vi "1. VI PRINCIPAL DDP GPE.vi"() -> ()   [LabVIEW 2019]
panel:
  out "Timeout":bool
  in  "Stop Button":bool
  in  "Menú":enum32{"Edición", "Reporte"}(tab)
  in  "Tab Control":T1(tab)
  out "Horizontal Pointer Slide 1":dbl
  in  "Umbralado":dbl(slide) scale=0.0..255.0
  in  "Umbralado Invertido":dbl(slide) scale=0.0..255.0
  out "Umbralado Invertido 2":dbl
  in  "Prewitt":dbl(slide) scale=0.0..10.0
  in  "Sobel":dbl(slide) scale=0.0..255.0
  out "Sobel Ind":dbl
  out "Prewitt Ind":dbl
  out "Filtro 2 Ind":dbl
  out "Filtro 1 Ind":dbl
  in  "Filtro 2":dbl(slide) scale=0.0..10.0
  in  "Filtro 1":dbl(slide) scale=0.0..10.0
  in  "+":bool
  in  "-":bool
  out "+ 2":bool
  out "- 2":bool
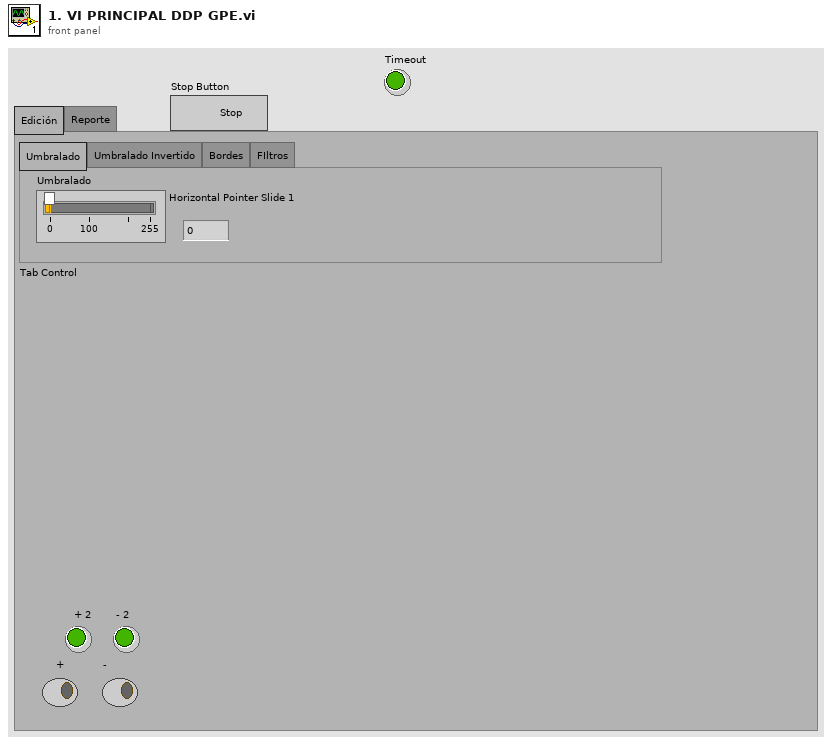
[diagram p1: front panel]
types:
  T1 = enum32{"Umbralado", "Umbralado Invertido", "Bordes", "FIltros"}
  T2 = cluster{"Umbralado":dbl, "Umbralado Invertido":dbl, "Filtro 1":dbl, "Filtro 2":dbl, "Sobel":dbl, "Prewitt":dbl}
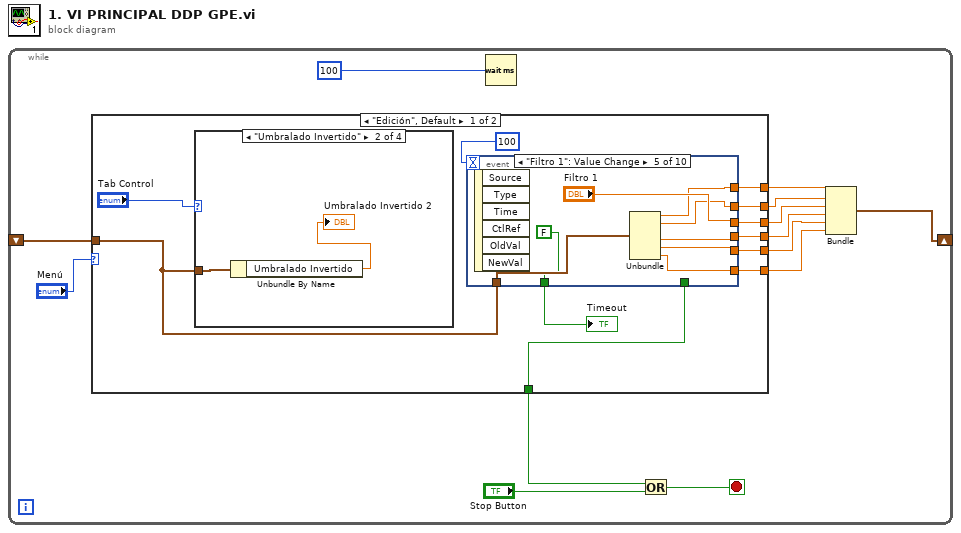
[diagram p0: block diagram]
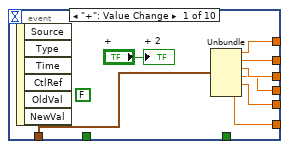
[diagram p2: hidden frame]
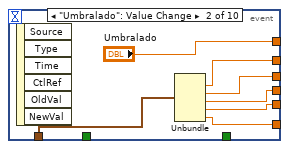
[diagram p3: hidden frame]
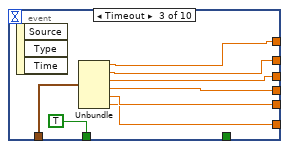
[diagram p4: hidden frame]
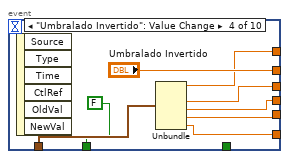
[diagram p5: hidden frame]
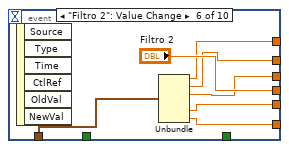
[diagram p6: hidden frame]
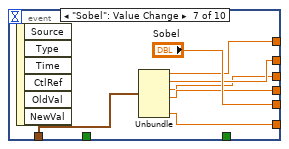
[diagram p7: hidden frame]
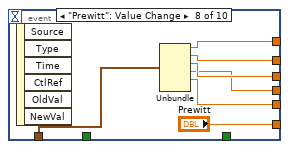
[diagram p8: hidden frame]
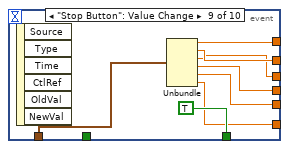
[diagram p9: hidden frame]
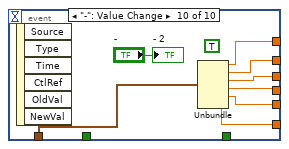
[diagram p10: hidden frame]
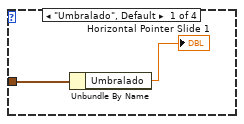
[diagram p11: hidden frame]
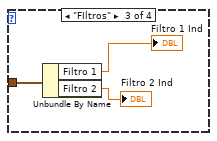
[diagram p12: hidden frame]
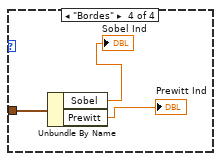
[diagram p13: hidden frame]
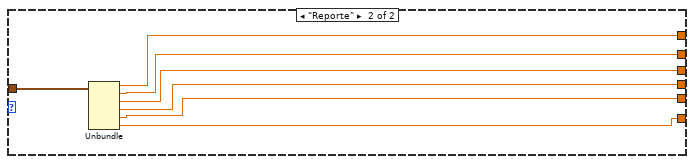
[diagram p14: hidden frame]
diagram:
  n1 = while {
    shift-right: [w5] -> _
    shift-left: _ -> [w8]
    stop <- w11 stop-if-true
    n2 = case shown="\"Edición\", Default" "Menú" {
      tunnel: [w23 _] -> w9
      tunnel: [w21 w115] -> w6
      tunnel: [w20 w116] -> w7
      tunnel: w8 -> [w15 w117]
      tunnel: [w19 w114] -> w4
      tunnel: [w18 w113] -> w3
      tunnel: [w17 w112] -> w2
      tunnel: [w16 w111] -> w1
      frame "Edición", Default {
        n3 = case shown="\"Umbralado Invertido\"" "Tab Control" {
          tunnel: w15 -> [w102 w104 w107 w110]
          frame "Umbralado", Default {
            n4 = Unbundle By Name(w102) -> ("Umbralado"=→"Horizontal Pointer Slide 1":dbl)
          }
          frame "Umbralado Invertido" {
            n5 = Unbundle By Name(w104) -> ("Umbralado Invertido"=→"Umbralado Invertido 2":dbl)
          }
          frame "FIltros" {
            n6 = Unbundle By Name(w107) -> ("Filtro 1"=→"Filtro 1 Ind":dbl, "Filtro 2"=→"Filtro 2 Ind":dbl)
          }
          frame "Bordes" {
            n7 = Unbundle By Name(w110) -> ("Sobel"=→"Sobel Ind":dbl, "Prewitt"=→"Prewitt Ind":dbl)
          }
        }
        n8 = event shown="[4] \"Filtro 1\": Value Change" {
          selector: _ -> [_ _ _ _ _ _ _ _ _ _]
          dyn-events: _ -> [_ _ _ _ _ _ _ _ _ _]
          timeout: 100 -> [_ _ _ _ _ _ _ _ _ _]
          tunnel: [_ _ _ _ _ _ _ _ TRUE _] -> w23
          tunnel: [w29 w37 w45 "Umbralado Invertido" w60 w67 w72 w81 w89 w97] -> w21
          tunnel: [w30 "Umbralado" w46 w53 w61 w68 w74 w82 w90 w98] -> w20
          tunnel: [w28 w36 w44 w52 "Filtro 1" w66 w71 w80 w88 w96] -> w19
          tunnel: [w27 w35 w43 w51 w59 "Filtro 2" w73 w79 w87 w95] -> w18
          tunnel: [w26 w34 w42 w50 w58 w65 "Sobel" w78 w86 w94] -> w17
          tunnel: [w25 w33 w41 w49 w57 w64 w75 "Prewitt" w85 w93] -> w16
          tunnel: w15 -> [w31 w38 w47 w54 w62 w69 w76 w83 w91 w99]
          tunnel: [_ _ TRUE ("Timeout") FALSE FALSE _ _ _ _ _] -> w14
          event "+": Value Change {
            (unwired) FALSE
            n9 = event-data() -> ()  [unwired: 1 in, 6 out]
            n10 = Unbundle(w31) -> ("Umbralado"=w30:dbl, "Umbralado Invertido"=w29:dbl, "Filtro 1"=w28:dbl, "Filtro 2"=w27:dbl, "Sobel"=w26:dbl, "Prewitt"=w25:dbl)
            "+ 2" <- "+"
          }
          event "Umbralado": Value Change {
            n11 = event-data() -> ()  [unwired: 1 in, 6 out]
            n12 = Unbundle(w38) -> ("Umbralado Invertido"=w37:dbl, "Filtro 1"=w36:dbl, "Filtro 2"=w35:dbl, "Sobel"=w34:dbl, "Prewitt"=w33:dbl)  [unwired: 1 out]
          }
          event Timeout {
            n13 = event-data() -> ()  [unwired: 1 in, 3 out]
            n14 = Unbundle(w47) -> ("Umbralado"=w46:dbl, "Umbralado Invertido"=w45:dbl, "Filtro 1"=w44:dbl, "Filtro 2"=w43:dbl, "Sobel"=w42:dbl, "Prewitt"=w41:dbl)
          }
          event "Umbralado Invertido": Value Change {
            n15 = event-data() -> ()  [unwired: 1 in, 6 out]
            n16 = Unbundle(w54) -> ("Umbralado"=w53:dbl, "Filtro 1"=w52:dbl, "Filtro 2"=w51:dbl, "Sobel"=w50:dbl, "Prewitt"=w49:dbl)  [unwired: 1 out]
          }
          event "Filtro 1": Value Change {
            n17 = event-data() -> ()  [unwired: 1 in, 6 out]
            n18 = Unbundle(w62) -> ("Umbralado"=w61:dbl, "Umbralado Invertido"=w60:dbl, "Filtro 2"=w59:dbl, "Sobel"=w58:dbl, "Prewitt"=w57:dbl)  [unwired: 1 out]
          }
          event "Filtro 2": Value Change {
            n19 = event-data() -> ()  [unwired: 1 in, 6 out]
            n20 = Unbundle(w69) -> ("Umbralado"=w68:dbl, "Umbralado Invertido"=w67:dbl, "Filtro 1"=w66:dbl, "Sobel"=w65:dbl, "Prewitt"=w64:dbl)  [unwired: 1 out]
          }
          event "Sobel": Value Change {
            n21 = event-data() -> ()  [unwired: 1 in, 6 out]
            n22 = Unbundle(w76) -> ("Umbralado"=w74:dbl, "Umbralado Invertido"=w72:dbl, "Filtro 1"=w71:dbl, "Filtro 2"=w73:dbl, "Prewitt"=w75:dbl)  [unwired: 1 out]
          }
          event "Prewitt": Value Change {
            n23 = event-data() -> ()  [unwired: 1 in, 6 out]
            n24 = Unbundle(w83) -> ("Umbralado"=w82:dbl, "Umbralado Invertido"=w81:dbl, "Filtro 1"=w80:dbl, "Filtro 2"=w79:dbl, "Sobel"=w78:dbl)  [unwired: 1 out]
          }
          event "Stop Button": Value Change {
            n25 = event-data() -> ()  [unwired: 1 in, 6 out]
            n26 = Unbundle(w91) -> ("Umbralado"=w90:dbl, "Umbralado Invertido"=w89:dbl, "Filtro 1"=w88:dbl, "Filtro 2"=w87:dbl, "Sobel"=w86:dbl, "Prewitt"=w85:dbl)
          }
          event "-": Value Change {
            (unwired) TRUE
            n27 = event-data() -> ()  [unwired: 1 in, 6 out]
            n28 = Unbundle(w99) -> ("Umbralado"=w98:dbl, "Umbralado Invertido"=w97:dbl, "Filtro 1"=w96:dbl, "Filtro 2"=w95:dbl, "Sobel"=w94:dbl, "Prewitt"=w93:dbl)
            "- 2" <- "-"
          }
        }
        "Timeout" <- w14
      }
      frame "Reporte" {
        n29 = Unbundle(w117) -> ("Umbralado"=w116:dbl, "Umbralado Invertido"=w115:dbl, "Filtro 1"=w114:dbl, "Filtro 2"=w113:dbl, "Sobel"=w112:dbl, "Prewitt"=w111:dbl)
      }
    }
    n30 = Wait (ms)(milliseconds to wait=u32 100) -> ()  [unwired: 1 out]
    n31 = Or(x=w9, y="Stop Button") -> (x .or. y?=w11:bool)
    n32 = Bundle("Umbralado"=w7, "Umbralado Invertido"=w6, "Filtro 1"=w4, "Filtro 2"=w3, "Sobel"=w2, "Prewitt"=w1) -> (w5:T2)  [unwired: 1 in]
  }
